vi "SVT Audio Filter.vi"   [LabVIEW 2017, in "SoundVib_AudioFilter.lvlib"]
doc: "Applies the selected audio weighting filter to the <B>scaled signal [EU]</B>. Wire data to the <B>scaled signal [EU]</B> input to determine the polymorphic instance to use or manually select the instance."
uses:
  <vilib>/addons/Sound and Vibration/svt_Weighting/SoundVib_AudioFilter.lvlib
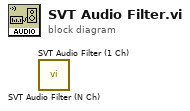
[diagram p0: block diagram]
diagram:
  n1 = call <vilib>:"SVT Audio Filter (N Ch).vi"() -> ()  [unwired: 8 in, 4 out]
  n2 = call <vilib>:"SVT Audio Filter (1 Ch).vi"() -> ()  [unwired: 8 in, 4 out]
